vi "JAUS Header Encoder.vi"(1 "Message Type (0-5)":u8, 2 "HC flags (6-7)":u8, 3 "Data Size (8-23)":u16, 4 "HC Number (24-31)":u8, 6 "HC Length (32-39)":u8, 8 "Priority(40-41)":u8, 10 "Broadcast Flags (42-43)":u8, 11 "Payload":string, 12 "Source ID (80-95)":u32 format="%x", 13 "Destination ID (48-79)":u32 format="%x", 14 "Data Flags (46-47)":u8, 15 "Ack/Nak (44-45)":u8) -> (0 "Encoded JAUS Message":string)   [LabVIEW 2009]
uses:
  cRIO/Functional Global Variables/Actions for FG's.ctl
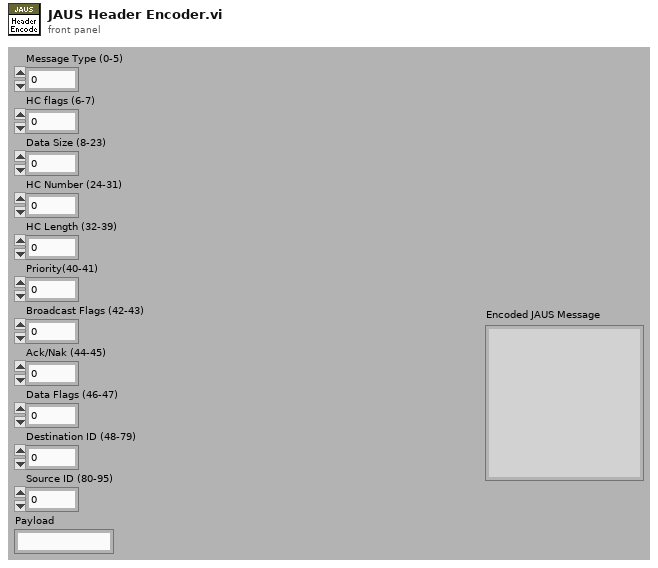
[diagram p1: front panel]
types:
  T1 = typedef "Actions for FG's.ctl" = enum16{"Read", "Write"}
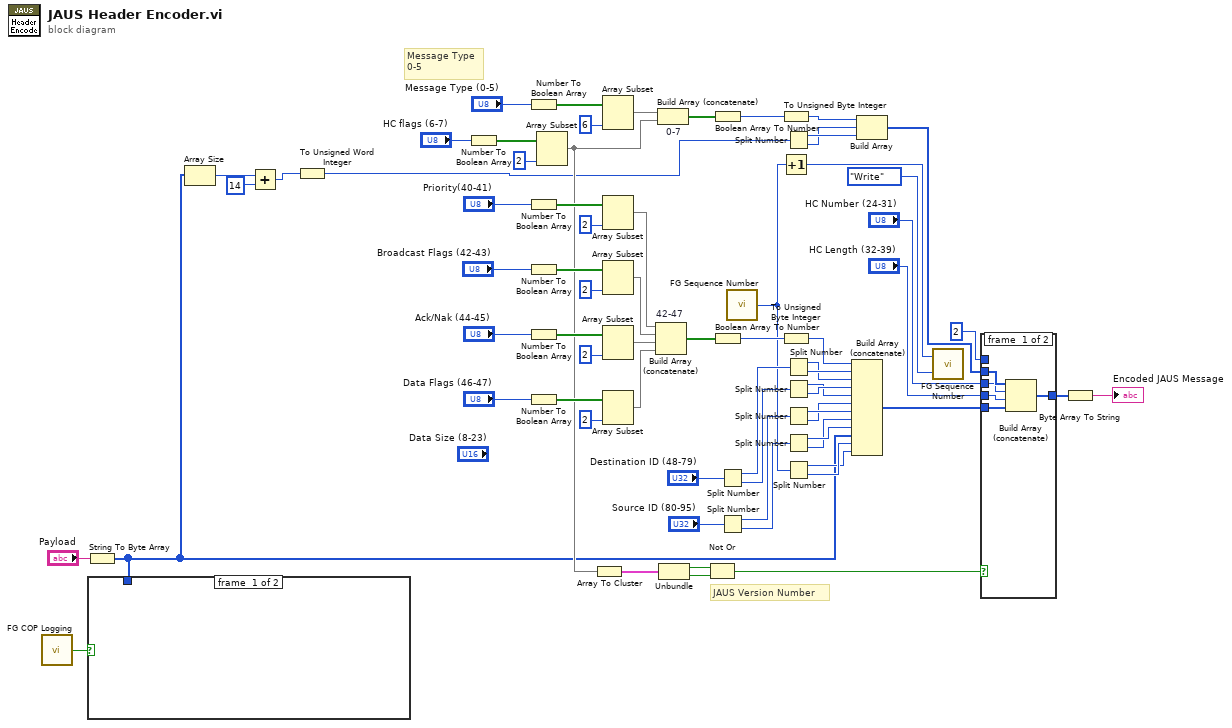
[diagram p0: block diagram]
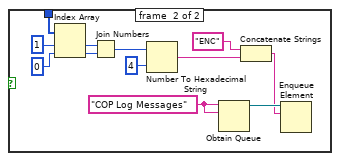
[diagram p2: hidden frame]
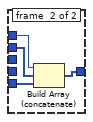
[diagram p3: hidden frame]
diagram:
  # "JAUS Version Number"
  # "Message Type\n0-5"
  n1 = call "FG COP Logging.vi"() -> ("Logging? out"=w1:bool)  [unwired: 2 in]
  n2 = String To Byte Array(string="Payload") -> (unsigned byte array=w2:u8[])
  n3 = case shown="True" w1 {
    tunnel: w2 -> [_ w81]
    frame #0 {
    }
    frame #1 {
      w74 = "COP Log Messages" ("name (unnamed)")
      n4 = Index Array(array=w81, index #1=1 ("index"), index #2=0 ("index")) -> (element #1=w77:u8, element #2=w78:u8)
      n5 = Join Numbers(hi=w77, lo=w78) -> ((hi.lo)=w75:u16)
      n6 = Number To Hexadecimal String(1:i16 4 ("width (-)"), 2:w75) -> (0:w73:string)
      n7 = Obtain Queue(name (unnamed)=w74, element data type=w74) -> (queue out=w72:refnum<queue>)  [unwired: 3 in, 2 out]
      n8 = Concatenate Strings("ENC" ("string"), w73) -> (w71:string)
      n9 = Enqueue Element(queue=w72, element=w71) -> ()  [unwired: 2 in, 3 out]
    }
  }
  n10 = Array Size(array=w2) -> (size(s)=w67:i32)
  n11 = Add(x=w67, y=14) -> (x+y=w65:i32)
  n12 = To Unsigned Word Integer(number=w65) -> (unsigned 16bit integer=w3:u16)
  n13 = Number To Boolean Array(number="HC flags (6-7)") -> (Boolean array=w60:bool[])
  n14 = Number To Boolean Array(number="Message Type (0-5)") -> (Boolean array=w62:bool[])
  n15 = Number To Boolean Array(number="Priority(40-41)") -> (Boolean array=w50:bool[])
  n16 = Number To Boolean Array(number="Broadcast Flags (42-43)") -> (Boolean array=w49:bool[])
  n17 = Number To Boolean Array(number="Ack/Nak (44-45)") -> (Boolean array=w48:bool[])
  n18 = Number To Boolean Array(number="Data Flags (46-47)") -> (Boolean array=w47:bool[])
  n19 = Array Subset(array=w60, length=2) -> (w28:bool[])  [unwired: 1 in]
  n20 = Array To Cluster(array=w28) -> (cluster=w27:cluster{"[0]":bool, "[1]":bool})
  n21 = Array Subset(array=w62, length=6) -> (w46:bool[])  [unwired: 1 in]
  n22 = Array Subset(array=w50, length=2) -> (w42:bool[])  [unwired: 1 in]
  n23 = Array Subset(array=w49, length=2) -> (w41:bool[])  [unwired: 1 in]
  n24 = Array Subset(array=w48, length=2) -> (w40:bool[])  [unwired: 1 in]
  n25 = Array Subset(array=w47, length=2) -> (w39:bool[])  [unwired: 1 in]
  n26 = Build Array (concatenate) "42-47"(w42, w41, w40, w39) -> (w38:bool[])
  n27 = Build Array (concatenate) "0-7"(w46, w28) -> (w45:bool[])
  n28 = Unbundle(w27) -> ("[0]"=w26:bool, "[1]"=w25:bool)
  n29 = Not Or(1:w25, 2:w26) -> (0:w29:bool)
  n30 = Boolean Array To Number(Boolean array=w45) -> (number=w37:u32)
  n31 = Boolean Array To Number(Boolean array=w38) -> (number=w36:u32)
  n32 = Split Number(x="Destination ID (48-79)") -> (hi(x)=w13:u16, lo(x)=w14:u16)
  n33 = Split Number(x="Source ID (80-95)") -> (hi(x)=w12:u16, lo(x)=w9:u16)
  n34 = call "FG Sequence Number.vi"() -> ("Sequence Number out"=w5:u16)  [unwired: 2 in]
  n35 = To Unsigned Byte Integer(number=w37) -> (unsigned 8bit integer=w34:u8)
  n36 = Increment(x=w5) -> (x+1=w4:u16)
  n37 = To Unsigned Byte Integer(number=w36) -> (unsigned 8bit integer=w35:u8)
  n38 = Split Number(x=w3) -> (hi(x)=w17:u8, lo(x)=w16:u8)
  n39 = Split Number(x=w13) -> (hi(x)=w20:u8, lo(x)=w21:u8)
  n40 = Split Number(x=w14) -> (hi(x)=w22:u8, lo(x)=w23:u8)
  n41 = Split Number(x=w12) -> (hi(x)=w11:u8, lo(x)=w10:u8)
  n42 = Split Number(x=w9) -> (hi(x)=w8:u8, lo(x)=w7:u8)
  n43 = Split Number(x=w5) -> (hi(x)=w18:u8, lo(x)=w19:u8)
  n44 = Build Array (concatenate)(w35, w21, w20, w23, w22, w10, w11, w7, w8, w2, w19, w18) -> (w24:u8[])
  n45 = Build Array(w34, w16, w17) -> (w32:u8[])
  n46 = call "FG Sequence Number.vi"("FG Action (Read)"=Actions_for_FG's."Write", "Sequence Number in"=w4) -> ()  [unwired: 1 out]
  n47 = case shown="False" w29 {
    tunnel: [w86 w88] -> w33
    tunnel: w32 -> [w85 w90]
    tunnel: w24 -> [w84 w89]
    tunnel: "HC Length (32-39)" -> [w83 _]
    tunnel: "HC Number (24-31)" -> [w82 _]
    tunnel: u8 2 ("Source ID (80-95)") -> [_ w87]
    frame #0 {
      n48 = Build Array (concatenate)(w85, w82, w83, w84) -> (w86:u8[])
    }
    frame #1 {
      n49 = Build Array (concatenate)(w87, w90, w89) -> (w88:u8[])
    }
  }
  n50 = Byte Array To String(unsigned byte array=w33) -> (string=→"Encoded JAUS Message":string)
